vi "Lasers monitor.vi"(0 "Update interval (ms)":u32=1000, 1 "Stop monitor":bool) -> (2 "GREEN LASER":T1, 3 "BLUE LASER":T1, 4 "Initialisation error":errorcluster, 5 "IO error (first)":errorcluster)   [LabVIEW 2014]
uses:
  Monitor values.ctl
  Laser enum.ctl
  Commands.ctl
panel:
  out "Second harmonic generator temperature":T2(graph)
  out "Birefringent filter temperature":T2(graph)
  out "Thermoelectric cooler temperature":T2(graph)
  out "Thermoelectric drive voltage":T2(graph)
  out "Laser diode drive current":T2(graph)
  out "Laser light power":T2(graph)
  # "PN 05/11/2014"
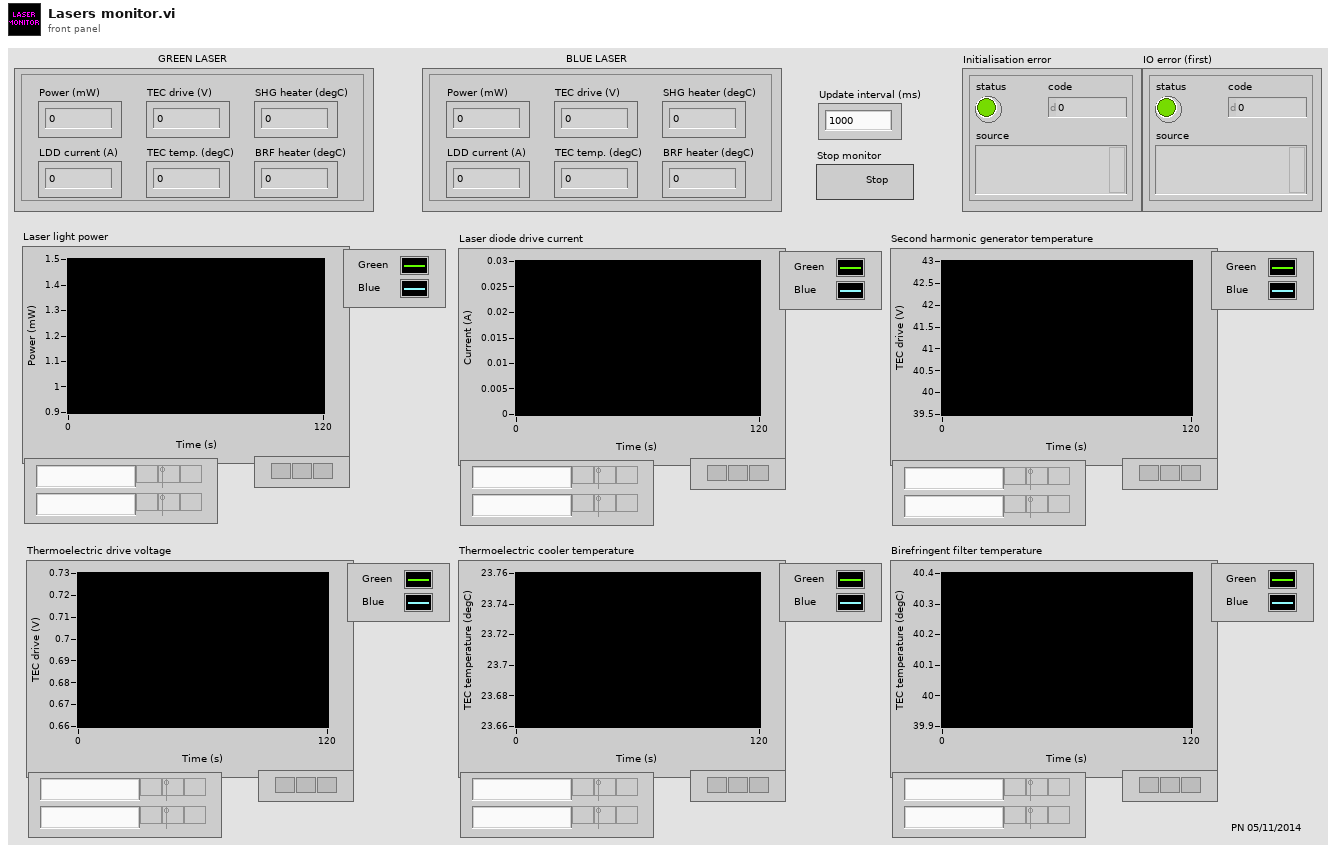
[diagram p1: front panel]
types:
  T1 = typedef "Monitor values.ctl" = cluster{"Power (mW)":sgl, "LDD current (A)":sgl, "TEC drive (V)":sgl, "TEC temp. (degC)":sgl, "SHG heater (degC)":sgl, "BRF heater (degC)":sgl}
  T2 = cluster{"response value":sgl, "response value":sgl}
  T3 = typedef "Commands.ctl" = u8
  T4 = typedef "Laser enum.ctl" = u8
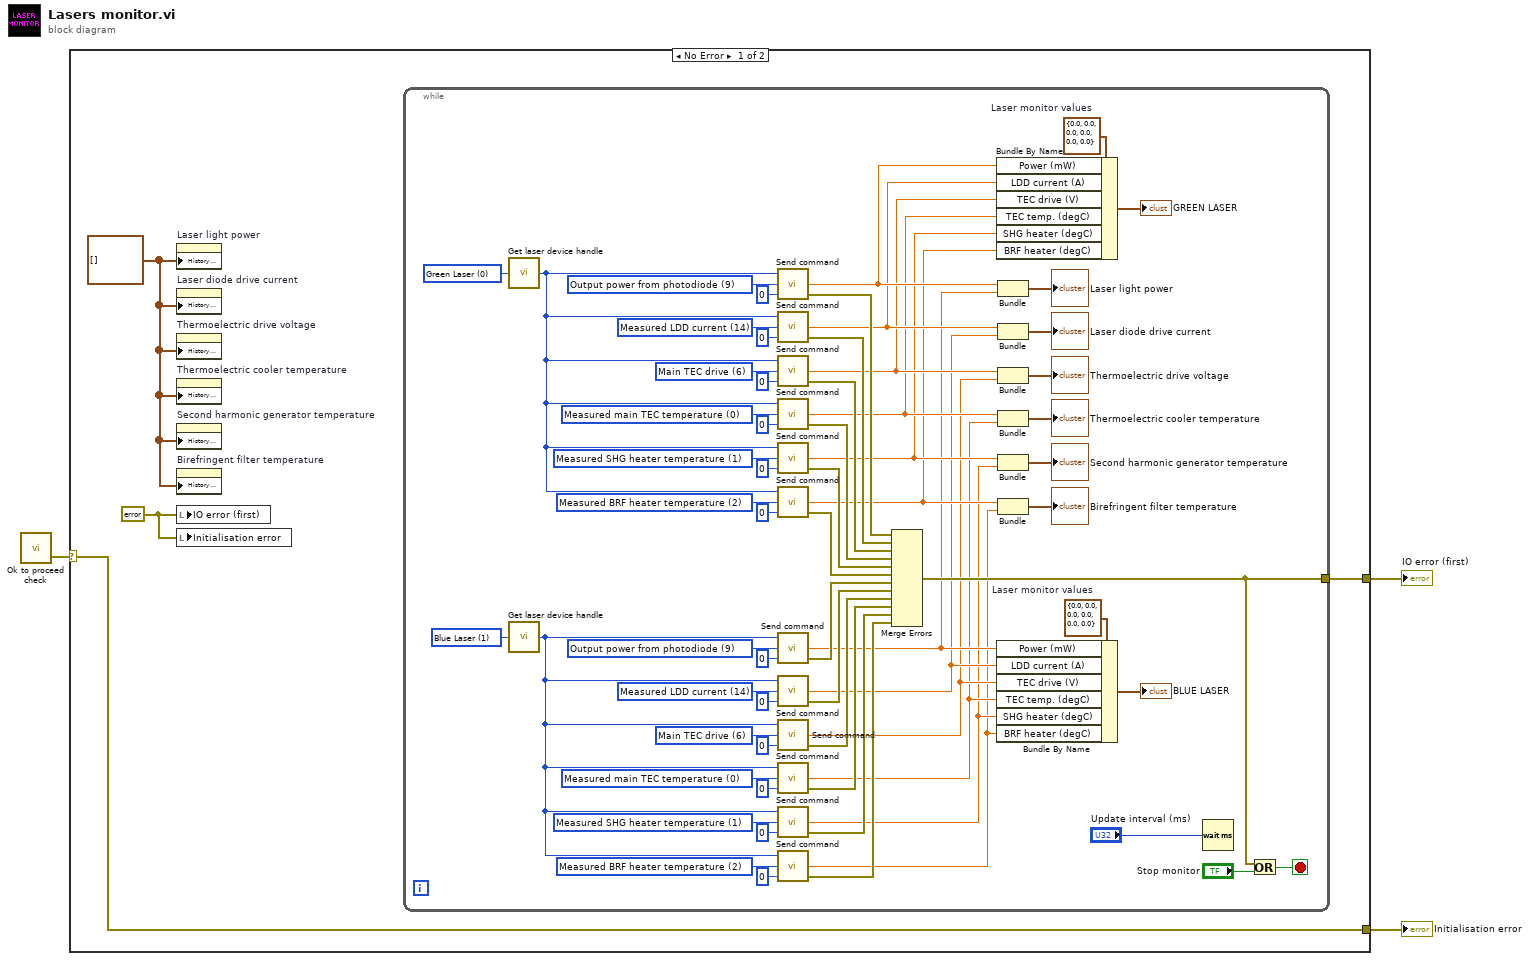
[diagram p0: block diagram]
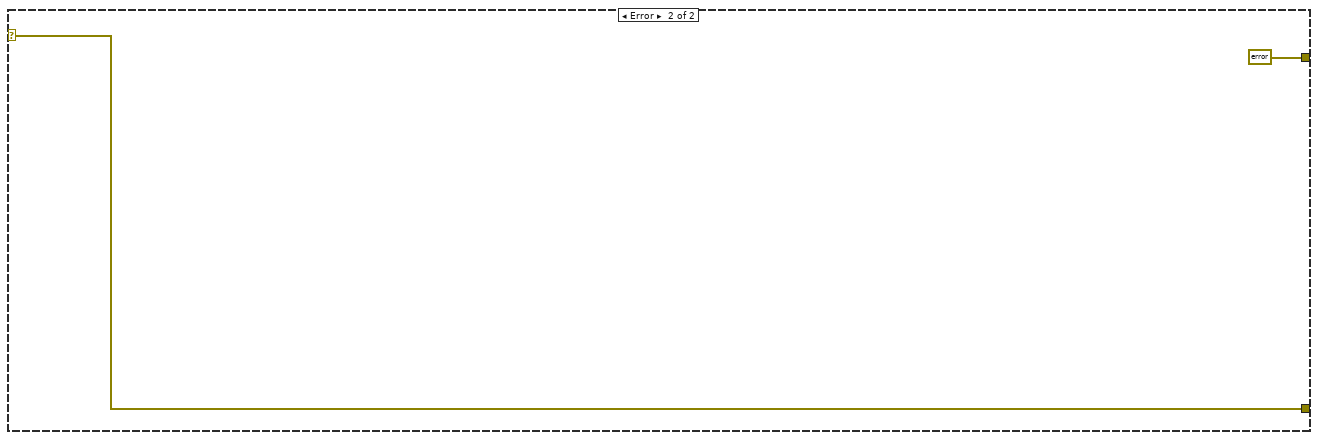
[diagram p2: hidden frame]
diagram:
  n1 = call "Ok to proceed check.vi"() -> ("Error"=w3:errorcluster)  [unwired: 2 in, 1 out]
  n2 = case shown="No Error" w3 {
    selector: w3 -> [w7 w75]
    tunnel: [w7 w75] -> w2
    tunnel: [w6 errorcluster {"status"=FALSE, "code"=0, "source"=""} ("error IO")] -> w1
    frame No Error {
      w4 = errorcluster {"status"=FALSE, "code"=0, "source"=""} ("IO error (first)")
      w5 = cluster{sgl, dbl}[] [] ("History Data")
      n3 = property on="Laser light power" class="WFChart (strict)"("History Data"=w5) -> ()  [unwired: 2 in, 2 out]
      n4 = property on="Laser diode drive current" class="WFChart (strict)"("History Data"=w5) -> ()  [unwired: 2 in, 2 out]
      n5 = property on="Thermoelectric drive voltage" class="WFChart (strict)"("History Data"=w5) -> ()  [unwired: 2 in, 2 out]
      n6 = property on="Thermoelectric cooler temperature" class="WFChart (strict)"("History Data"=w5) -> ()  [unwired: 2 in, 2 out]
      n7 = property on="Second harmonic generator temperature" class="WFChart (strict)"("History Data"=w5) -> ()  [unwired: 2 in, 2 out]
      n8 = property on="Birefringent filter temperature" class="WFChart (strict)"("History Data"=w5) -> ()  [unwired: 2 in, 2 out]
      n9 = local write "IO error (first)"(w4) -> ()
      n10 = local write "Initialisation error"(w4) -> ()
      n11 = while {
        tunnel: [w40] -> w6
        stop <- w41 stop-if-true
        w8 = T1 {"Power (mW)"=0.0, "LDD current (A)"=0.0, "TEC drive (V)"=0.0, "TEC temp. (degC)"=0.0, "SHG heater (degC)"=0.0, "BRF heater (degC)"=0.0}  # Laser monitor values
        w15 = T1 {"Power (mW)"=0.0, "LDD current (A)"=0.0, "TEC drive (V)"=0.0, "TEC temp. (degC)"=0.0, "SHG heater (degC)"=0.0, "BRF heater (degC)"=0.0}  # Laser monitor values
        w31 = T3 2 items=["Measured main TEC temperature"=0, "Measured SHG heater temperature"=1, "Measured BRF heater temperature"=2, "Main TEC temperature command"=3, "SHG heater temperature command"=4, "BRF heater temperature command"=5, "Main TEC drive"=6, "SHG heater drive"=7, "BRF heater drive"=8, "Output power from photodiode"=9, "Output power setpoint (Get)"=10, "Output power setpoint (Set)"=11, "Start-up power setting (Get)"=12, "Start-up power setting (Set)"=13, "Measured LDD current"=14, "Maximum LDD current limit"=15, "16-bit fault code"=16, "Head serial number"=17, "Head board rev"=18, "Head type"=19, "LDD enable state"=20, "Key switch command (Get)"=24, "Key switch command (Set)"=25, "Key switch actual"=26, "Interlock status"=27, "Head hours"=28, "Photo or current mode command (Get)"=29, "Photo or current mode command (Set)"=30, "Photo or current mode actual"=31, "Analog input enable command (Get)"=32, "Analog input enable command (Set)"=33, "Analog input actual"=34, "Power supply glue input"=36, "Power supply glue output"=37] ("Command")
        w30 = T3 1 items=["Measured main TEC temperature"=0, "Measured SHG heater temperature"=1, "Measured BRF heater temperature"=2, "Main TEC temperature command"=3, "SHG heater temperature command"=4, "BRF heater temperature command"=5, "Main TEC drive"=6, "SHG heater drive"=7, "BRF heater drive"=8, "Output power from photodiode"=9, "Output power setpoint (Get)"=10, "Output power setpoint (Set)"=11, "Start-up power setting (Get)"=12, "Start-up power setting (Set)"=13, "Measured LDD current"=14, "Maximum LDD current limit"=15, "16-bit fault code"=16, "Head serial number"=17, "Head board rev"=18, "Head type"=19, "LDD enable state"=20, "Key switch command (Get)"=24, "Key switch command (Set)"=25, "Key switch actual"=26, "Interlock status"=27, "Head hours"=28, "Photo or current mode command (Get)"=29, "Photo or current mode command (Set)"=30, "Photo or current mode actual"=31, "Analog input enable command (Get)"=32, "Analog input enable command (Set)"=33, "Analog input actual"=34, "Power supply glue input"=36, "Power supply glue output"=37] ("Command")
        w37 = T3 2 items=["Measured main TEC temperature"=0, "Measured SHG heater temperature"=1, "Measured BRF heater temperature"=2, "Main TEC temperature command"=3, "SHG heater temperature command"=4, "BRF heater temperature command"=5, "Main TEC drive"=6, "SHG heater drive"=7, "BRF heater drive"=8, "Output power from photodiode"=9, "Output power setpoint (Get)"=10, "Output power setpoint (Set)"=11, "Start-up power setting (Get)"=12, "Start-up power setting (Set)"=13, "Measured LDD current"=14, "Maximum LDD current limit"=15, "16-bit fault code"=16, "Head serial number"=17, "Head board rev"=18, "Head type"=19, "LDD enable state"=20, "Key switch command (Get)"=24, "Key switch command (Set)"=25, "Key switch actual"=26, "Interlock status"=27, "Head hours"=28, "Photo or current mode command (Get)"=29, "Photo or current mode command (Set)"=30, "Photo or current mode actual"=31, "Analog input enable command (Get)"=32, "Analog input enable command (Set)"=33, "Analog input actual"=34, "Power supply glue input"=36, "Power supply glue output"=37] ("Command")
        w38 = T3 1 items=["Measured main TEC temperature"=0, "Measured SHG heater temperature"=1, "Measured BRF heater temperature"=2, "Main TEC temperature command"=3, "SHG heater temperature command"=4, "BRF heater temperature command"=5, "Main TEC drive"=6, "SHG heater drive"=7, "BRF heater drive"=8, "Output power from photodiode"=9, "Output power setpoint (Get)"=10, "Output power setpoint (Set)"=11, "Start-up power setting (Get)"=12, "Start-up power setting (Set)"=13, "Measured LDD current"=14, "Maximum LDD current limit"=15, "16-bit fault code"=16, "Head serial number"=17, "Head board rev"=18, "Head type"=19, "LDD enable state"=20, "Key switch command (Get)"=24, "Key switch command (Set)"=25, "Key switch actual"=26, "Interlock status"=27, "Head hours"=28, "Photo or current mode command (Get)"=29, "Photo or current mode command (Set)"=30, "Photo or current mode actual"=31, "Analog input enable command (Get)"=32, "Analog input enable command (Set)"=33, "Analog input actual"=34, "Power supply glue input"=36, "Power supply glue output"=37] ("Command")
        w64 = T3 14 items=["Measured main TEC temperature"=0, "Measured SHG heater temperature"=1, "Measured BRF heater temperature"=2, "Main TEC temperature command"=3, "SHG heater temperature command"=4, "BRF heater temperature command"=5, "Main TEC drive"=6, "SHG heater drive"=7, "BRF heater drive"=8, "Output power from photodiode"=9, "Output power setpoint (Get)"=10, "Output power setpoint (Set)"=11, "Start-up power setting (Get)"=12, "Start-up power setting (Set)"=13, "Measured LDD current"=14, "Maximum LDD current limit"=15, "16-bit fault code"=16, "Head serial number"=17, "Head board rev"=18, "Head type"=19, "LDD enable state"=20, "Key switch command (Get)"=24, "Key switch command (Set)"=25, "Key switch actual"=26, "Interlock status"=27, "Head hours"=28, "Photo or current mode command (Get)"=29, "Photo or current mode command (Set)"=30, "Photo or current mode actual"=31, "Analog input enable command (Get)"=32, "Analog input enable command (Set)"=33, "Analog input actual"=34, "Power supply glue input"=36, "Power supply glue output"=37] ("Command")
        w61 = T3 0 items=["Measured main TEC temperature"=0, "Measured SHG heater temperature"=1, "Measured BRF heater temperature"=2, "Main TEC temperature command"=3, "SHG heater temperature command"=4, "BRF heater temperature command"=5, "Main TEC drive"=6, "SHG heater drive"=7, "BRF heater drive"=8, "Output power from photodiode"=9, "Output power setpoint (Get)"=10, "Output power setpoint (Set)"=11, "Start-up power setting (Get)"=12, "Start-up power setting (Set)"=13, "Measured LDD current"=14, "Maximum LDD current limit"=15, "16-bit fault code"=16, "Head serial number"=17, "Head board rev"=18, "Head type"=19, "LDD enable state"=20, "Key switch command (Get)"=24, "Key switch command (Set)"=25, "Key switch actual"=26, "Interlock status"=27, "Head hours"=28, "Photo or current mode command (Get)"=29, "Photo or current mode command (Set)"=30, "Photo or current mode actual"=31, "Analog input enable command (Get)"=32, "Analog input enable command (Set)"=33, "Analog input actual"=34, "Power supply glue input"=36, "Power supply glue output"=37] ("Command")
        w60 = T3 6 items=["Measured main TEC temperature"=0, "Measured SHG heater temperature"=1, "Measured BRF heater temperature"=2, "Main TEC temperature command"=3, "SHG heater temperature command"=4, "BRF heater temperature command"=5, "Main TEC drive"=6, "SHG heater drive"=7, "BRF heater drive"=8, "Output power from photodiode"=9, "Output power setpoint (Get)"=10, "Output power setpoint (Set)"=11, "Start-up power setting (Get)"=12, "Start-up power setting (Set)"=13, "Measured LDD current"=14, "Maximum LDD current limit"=15, "16-bit fault code"=16, "Head serial number"=17, "Head board rev"=18, "Head type"=19, "LDD enable state"=20, "Key switch command (Get)"=24, "Key switch command (Set)"=25, "Key switch actual"=26, "Interlock status"=27, "Head hours"=28, "Photo or current mode command (Get)"=29, "Photo or current mode command (Set)"=30, "Photo or current mode actual"=31, "Analog input enable command (Get)"=32, "Analog input enable command (Set)"=33, "Analog input actual"=34, "Power supply glue input"=36, "Power supply glue output"=37] ("Command")
        w57 = T3 9 items=["Measured main TEC temperature"=0, "Measured SHG heater temperature"=1, "Measured BRF heater temperature"=2, "Main TEC temperature command"=3, "SHG heater temperature command"=4, "BRF heater temperature command"=5, "Main TEC drive"=6, "SHG heater drive"=7, "BRF heater drive"=8, "Output power from photodiode"=9, "Output power setpoint (Get)"=10, "Output power setpoint (Set)"=11, "Start-up power setting (Get)"=12, "Start-up power setting (Set)"=13, "Measured LDD current"=14, "Maximum LDD current limit"=15, "16-bit fault code"=16, "Head serial number"=17, "Head board rev"=18, "Head type"=19, "LDD enable state"=20, "Key switch command (Get)"=24, "Key switch command (Set)"=25, "Key switch actual"=26, "Interlock status"=27, "Head hours"=28, "Photo or current mode command (Get)"=29, "Photo or current mode command (Set)"=30, "Photo or current mode actual"=31, "Analog input enable command (Get)"=32, "Analog input enable command (Set)"=33, "Analog input actual"=34, "Power supply glue input"=36, "Power supply glue output"=37] ("Command")
        w56 = T4 1 items=["Green Laser", "Blue Laser"] ("Selected laser")
        w65 = T3 14 items=["Measured main TEC temperature"=0, "Measured SHG heater temperature"=1, "Measured BRF heater temperature"=2, "Main TEC temperature command"=3, "SHG heater temperature command"=4, "BRF heater temperature command"=5, "Main TEC drive"=6, "SHG heater drive"=7, "BRF heater drive"=8, "Output power from photodiode"=9, "Output power setpoint (Get)"=10, "Output power setpoint (Set)"=11, "Start-up power setting (Get)"=12, "Start-up power setting (Set)"=13, "Measured LDD current"=14, "Maximum LDD current limit"=15, "16-bit fault code"=16, "Head serial number"=17, "Head board rev"=18, "Head type"=19, "LDD enable state"=20, "Key switch command (Get)"=24, "Key switch command (Set)"=25, "Key switch actual"=26, "Interlock status"=27, "Head hours"=28, "Photo or current mode command (Get)"=29, "Photo or current mode command (Set)"=30, "Photo or current mode actual"=31, "Analog input enable command (Get)"=32, "Analog input enable command (Set)"=33, "Analog input actual"=34, "Power supply glue input"=36, "Power supply glue output"=37] ("Command")
        w68 = T3 0 items=["Measured main TEC temperature"=0, "Measured SHG heater temperature"=1, "Measured BRF heater temperature"=2, "Main TEC temperature command"=3, "SHG heater temperature command"=4, "BRF heater temperature command"=5, "Main TEC drive"=6, "SHG heater drive"=7, "BRF heater drive"=8, "Output power from photodiode"=9, "Output power setpoint (Get)"=10, "Output power setpoint (Set)"=11, "Start-up power setting (Get)"=12, "Start-up power setting (Set)"=13, "Measured LDD current"=14, "Maximum LDD current limit"=15, "16-bit fault code"=16, "Head serial number"=17, "Head board rev"=18, "Head type"=19, "LDD enable state"=20, "Key switch command (Get)"=24, "Key switch command (Set)"=25, "Key switch actual"=26, "Interlock status"=27, "Head hours"=28, "Photo or current mode command (Get)"=29, "Photo or current mode command (Set)"=30, "Photo or current mode actual"=31, "Analog input enable command (Get)"=32, "Analog input enable command (Set)"=33, "Analog input actual"=34, "Power supply glue input"=36, "Power supply glue output"=37] ("Command")
        w69 = T3 6 items=["Measured main TEC temperature"=0, "Measured SHG heater temperature"=1, "Measured BRF heater temperature"=2, "Main TEC temperature command"=3, "SHG heater temperature command"=4, "BRF heater temperature command"=5, "Main TEC drive"=6, "SHG heater drive"=7, "BRF heater drive"=8, "Output power from photodiode"=9, "Output power setpoint (Get)"=10, "Output power setpoint (Set)"=11, "Start-up power setting (Get)"=12, "Start-up power setting (Set)"=13, "Measured LDD current"=14, "Maximum LDD current limit"=15, "16-bit fault code"=16, "Head serial number"=17, "Head board rev"=18, "Head type"=19, "LDD enable state"=20, "Key switch command (Get)"=24, "Key switch command (Set)"=25, "Key switch actual"=26, "Interlock status"=27, "Head hours"=28, "Photo or current mode command (Get)"=29, "Photo or current mode command (Set)"=30, "Photo or current mode actual"=31, "Analog input enable command (Get)"=32, "Analog input enable command (Set)"=33, "Analog input actual"=34, "Power supply glue input"=36, "Power supply glue output"=37] ("Command")
        w72 = T3 9 items=["Measured main TEC temperature"=0, "Measured SHG heater temperature"=1, "Measured BRF heater temperature"=2, "Main TEC temperature command"=3, "SHG heater temperature command"=4, "BRF heater temperature command"=5, "Main TEC drive"=6, "SHG heater drive"=7, "BRF heater drive"=8, "Output power from photodiode"=9, "Output power setpoint (Get)"=10, "Output power setpoint (Set)"=11, "Start-up power setting (Get)"=12, "Start-up power setting (Set)"=13, "Measured LDD current"=14, "Maximum LDD current limit"=15, "16-bit fault code"=16, "Head serial number"=17, "Head board rev"=18, "Head type"=19, "LDD enable state"=20, "Key switch command (Get)"=24, "Key switch command (Set)"=25, "Key switch actual"=26, "Interlock status"=27, "Head hours"=28, "Photo or current mode command (Get)"=29, "Photo or current mode command (Set)"=30, "Photo or current mode actual"=31, "Analog input enable command (Get)"=32, "Analog input enable command (Set)"=33, "Analog input actual"=34, "Power supply glue input"=36, "Power supply glue output"=37] ("Command")
        w73 = T4 0 items=["Green Laser", "Blue Laser"] ("Selected laser")
        n12 = call "Get laser device handle.vi"("Selected laser"=w73) -> ("Device handle"=w35:u32)
        n13 = call "Get laser device handle.vi"("Selected laser"=w56) -> ("Device handle"=w28:u32)
        n14 = call "Send command.vi"("Value"=u16 0, "Command"=w72, "Device handle"=w35) -> ("Error"=w50:errorcluster, "response value"=w23:sgl)  [unwired: 1 out]
        n15 = call "Send command.vi"("Value"=u16 0, "Command"=w65, "Device handle"=w35) -> ("Error"=w49:errorcluster, "response value"=w22:sgl)  [unwired: 1 out]
        n16 = call "Send command.vi"("Value"=u16 0, "Command"=w69, "Device handle"=w35) -> ("Error"=w48:errorcluster, "response value"=w21:sgl)  [unwired: 1 out]
        n17 = call "Send command.vi"("Value"=u16 0, "Command"=w68, "Device handle"=w35) -> ("Error"=w47:errorcluster, "response value"=w20:sgl)  [unwired: 1 out]
        n18 = call "Send command.vi"("Value"=u16 0, "Command"=w38, "Device handle"=w35) -> ("Error"=w34:errorcluster, "response value"=w19:sgl)  [unwired: 1 out]
        n19 = call "Send command.vi"("Value"=u16 0, "Command"=w37, "Device handle"=w35) -> ("Error"=w33:errorcluster, "response value"=w18:sgl)  [unwired: 1 out]
        n20 = call "Send command.vi"("Value"=u16 0, "Command"=w57, "Device handle"=w28) -> ("Error"=w46:errorcluster, "response value"=w14:sgl)  [unwired: 1 out]
        n21 = call "Send command.vi"("Value"=u16 0, "Command"=w64, "Device handle"=w28) -> ("Error"=w45:errorcluster, "response value"=w13:sgl)  [unwired: 1 out]
        n22 = call "Send command.vi"("Value"=u16 0, "Command"=w60, "Device handle"=w28) -> ("Error"=w44:errorcluster, "response value"=w12:sgl)  [unwired: 1 out]
        n23 = call "Send command.vi"("Value"=u16 0, "Command"=w61, "Device handle"=w28) -> ("Error"=w43:errorcluster, "response value"=w11:sgl)  [unwired: 1 out]
        n24 = call "Send command.vi"("Value"=u16 0, "Command"=w30, "Device handle"=w28) -> ("Error"=w27:errorcluster, "response value"=w10:sgl)  [unwired: 1 out]
        n25 = call "Send command.vi"("Value"=u16 0, "Command"=w31, "Device handle"=w28) -> ("Error"=w26:errorcluster, "response value"=w9:sgl)  [unwired: 1 out]
        n26 = Merge Errors(w50, w49, w48, w47, w34, w33, w46, w45, w44, w43, w27, w26) -> (w40:errorcluster)
        n27 = Bundle By Name(cluster=w15, "Power (mW)"=w23, "LDD current (A)"=w22, "TEC drive (V)"=w21, "TEC temp. (degC)"=w20, "SHG heater (degC)"=w19, "BRF heater (degC)"=w18) -> (→"GREEN LASER":T1)
        n28 = Bundle By Name(cluster=w8, "Power (mW)"=w14, "LDD current (A)"=w13, "TEC drive (V)"=w12, "TEC temp. (degC)"=w11, "SHG heater (degC)"=w10, "BRF heater (degC)"=w9) -> (→"BLUE LASER":T1)
        n29 = Bundle("response value"=w23, "response value"=w14) -> (→"Laser light power":T2)  [unwired: 1 in]
        n30 = Bundle("response value"=w22, "response value"=w13) -> (→"Laser diode drive current":T2)  [unwired: 1 in]
        n31 = Bundle("response value"=w21, "response value"=w12) -> (→"Thermoelectric drive voltage":T2)  [unwired: 1 in]
        n32 = Bundle("response value"=w20, "response value"=w11) -> (→"Thermoelectric cooler temperature":T2)  [unwired: 1 in]
        n33 = Bundle("response value"=w19, "response value"=w10) -> (→"Second harmonic generator temperature":T2)  [unwired: 1 in]
        n34 = Bundle("response value"=w18, "response value"=w9) -> (→"Birefringent filter temperature":T2)  [unwired: 1 in]
        n35 = Wait (ms)(milliseconds to wait="Update interval (ms)") -> ()  [unwired: 1 out]
        n36 = Or(x=w40, y="Stop monitor") -> (x .or. y?=w41:bool)
      }
    }
    frame Error {
    }
  }
  "Initialisation error" <- w2
  "IO error (first)" <- w1
